vi "Sample Push go for Push State.vi"(8 "error in (no error)":errorcluster, 11 "cRIO-CO2 in":refnum<class "cRIO-CO2.lvclass">) -> (0 "error out":errorcluster, 3 "cRIO-CO2 out":refnum<class "cRIO-CO2.lvclass">)   [LabVIEW 2015, in "cRIO-Carbondioxide.lvlib" / "cRIO-CO2.lvlib" / "cRIO-CO2.lvclass"]
uses:
  cRIO-CO2.lvclass
  cRIO-CO2.lvclass/cRIO-CO2.ctl
  Controls/Sample Push State Enumerator.ctl
  State Elapsed Time.vi
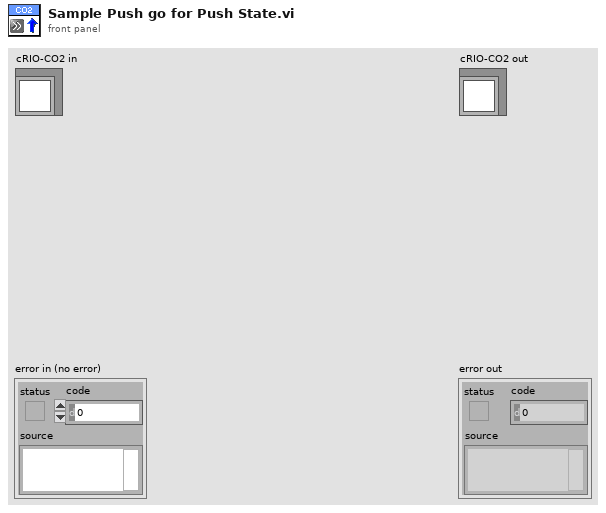
[diagram p1: front panel]
types:
  T1 = typedef "Sample Push State Enumerator.ctl" = enum16{"Undefined", "Initialize", "Dilute", "Close Transfer Line", "Start Heaters", "Warm Up Syringe", "Ready to Push", "Push", "Initiate Stash", "Stash", "Complete", "Abort", "Idle", "Error"}
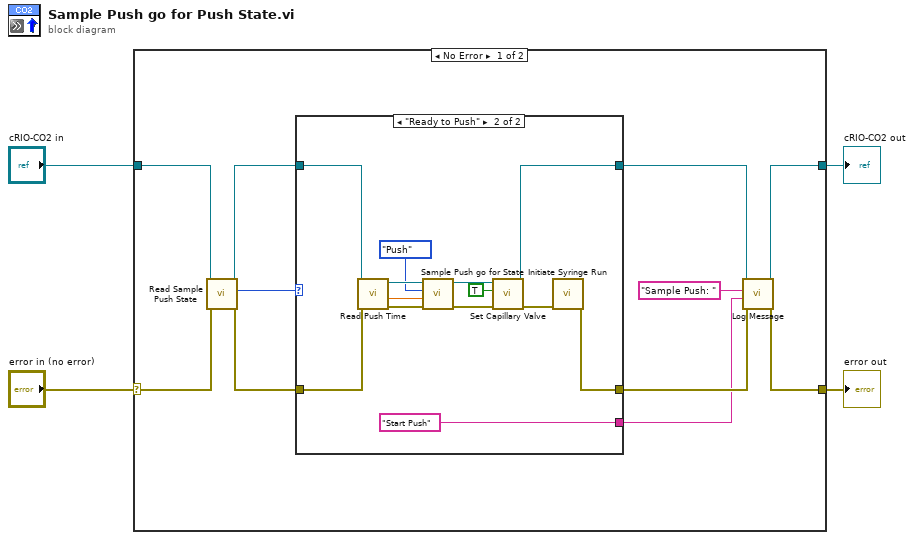
[diagram p0: block diagram]
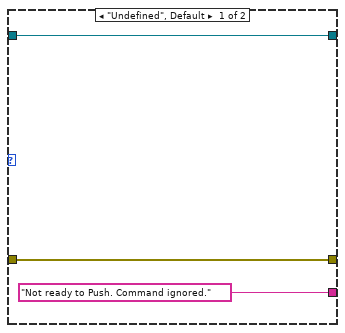
[diagram p2: hidden frame]
diagram:
  n1 = case shown="No Error" "error in (no error)" {
    selector: "error in (no error)" -> [w15 w33]
    tunnel: [w8 w33] -> w3
    tunnel: [w6 w32] -> w1
    tunnel: "cRIO-CO2 in" -> [w14 w32]
    frame No Error {
      n2 = call "Read Sample Push State.vi"("error in (no error)"=w15, "cRIO-CO2 in"=w14) -> ("error out"=w13:errorcluster, "Sample Push State"=w11:T1, "cRIO-CO2 out"=w12:refnum<class "cRIO-CO2.lvclass">)  [unwired: 3 in, 4 out]
      n3 = case shown="\"Ready to Push\"" w11 {
        tunnel: w13 -> [w17 w29]
        tunnel: [w17 w20] -> w9
        tunnel: w12 -> [w18 w31]
        tunnel: [w18 w22] -> w7
        tunnel: ["Not ready to Push. Command ignored." ("String") "Start Push" ("String")] -> w5
        frame "Undefined", Default {
        }
        frame "Ready to Push" {
          n4 = call "Read Push Time.vi"("error in (no error)"=w29, "cRIO-CO2 in"=w31) -> ("error out"=w28:errorcluster, "Push Time (sec)"=w27:dbl, "cRIO-CO2 out"=w30:refnum<class "cRIO-CO2.lvclass">)  [unwired: 7 in]
          n5 = call "Sample Push go for State.vi"("error in (no error)"=w28, "State Timeout (Inf=no timeout )"=w27, "Sample Push State"=Sample_Push_State_Enumerator."Push", "cRIO-CO2 in"=w30) -> ("error out"=w19:errorcluster, "cRIO-CO2 out"=w23:refnum<class "cRIO-CO2.lvclass">)  [unwired: 6 in]
          n6 = call "Set Capillary Valve.vi"("error in (no error)"=w19, "ON/OFF(OFF)"=TRUE, "cRIO-CO2 in"=w23) -> ("error out"=w21:errorcluster, "cRIO-CO2 out"=w22:refnum<class "cRIO-CO2.lvclass">)  [unwired: 7 in]
          n7 = call "Initiate Syringe Run.vi"("error in (no error)"=w21) -> ("error out"=w20:errorcluster)  [unwired: 10 in]
        }
      }
      n8 = call "Log Message.vi"("error in (no error)"=w9, "String"=w5, "Source Name"="Sample Push: ", "cRIO-CO2 in"=w7) -> ("error out"=w8:errorcluster, "cRIO-CO2 out"=w6:refnum<class "cRIO-CO2.lvclass">)  [unwired: 6 in]
    }
    frame Error {
    }
  }
  "error out" <- w3
  "cRIO-CO2 out" <- w1
